vi "Registry - unregister silences appender.vi"(8 "error in (no error)":errorcluster) -> (0 "error out":errorcluster)   [LabVIEW 2026, in "Tests.lvlib"]
doc: "Verifies that unregistering one appender stops its delivery while the others keep receiving. Registers three queue-mode relay appenders, logs once (all three receive), unregisters relayB, logs again, and asserts the two survivors receive the second message and relayB receives nothing. Exercises the IDAbsent barrier in UnregisterAppender."
uses:
  Tests.lvlib
  src/TypeDefs/Severity.ctl
  <vilib>/addons/_JKI Toolkits/Caraya/classes/Assert/Assert False.vi
  <vilib>/addons/_JKI Toolkits/Caraya/classes/Assert/Assert Equal Value_Variant.vi
  <vilib>/addons/_JKI Toolkits/Caraya/classes/Assert/Assert True.vi
  <vilib>/addons/_JKI Toolkits/Caraya/classes/Assert/Assert Not Error.vi
  <vilib>/addons/_JKI Toolkits/Caraya/classes/Test/Test.lvclass
  src/Lumberjack.lvlib
  src/Public/Logger.lvclass/Logger.lvclass
  <vilib>/addons/_JKI Toolkits/Caraya/classes/Assert/Assert.lvclass
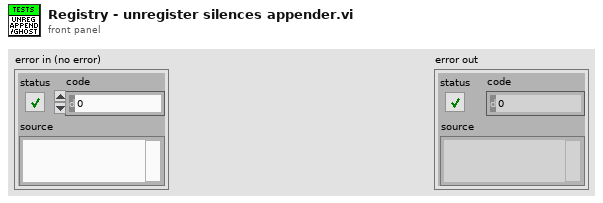
[diagram p1: front panel]
types:
  T1 = typedef "Lumberjack.lvlib/Severity.ctl" = enum16{"OFF", "FATAL", "ERROR", "WARN", "INFO", "DEBUG", "TRACE", "ALL"}
  T2 = typedef "Lumberjack.lvlib/Statement.ctl" = cluster{"timestamp":timestamp, "level":T1, "sourceTag":string, "originVI":string, "message":string}
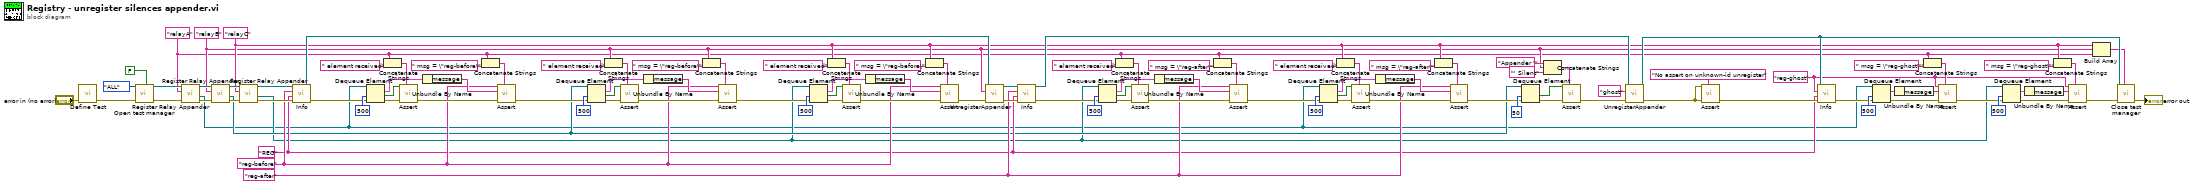
[diagram p0: block diagram]
diagram:
  w11 = "reg-ghost" ("message")
  w41 = "reg-after" ("message")
  w7 = "relayC"
  w6 = "relayB"
  w5 = "relayA"
  w27 = "REG" ("sourceTag")
  w68 = "reg-before" ("message")
  n1 = call <vilib>:"Define Test.vi"("error in (no error)"="error in (no error)") -> ("error out"=w111:errorcluster)  [unwired: 9 in, 1 out]
  n2 = call "Open test manager.vi"("enableDefaultFile"=FALSE, "error in (no error)"=w111, "globalThreshold"=Severity."ALL") -> ("error out"=w108:errorcluster, "Logger out"=w109:refnum<class "Logger.lvclass">)  [unwired: 7 in]
  n3 = call "Register Relay Appender.vi"("error in (no error)"=w108, "id in"=w5, "Logger in"=w109) -> ("error out"=w107:errorcluster, "relayQueue"=w3:refnum<queue>, "Logger out"=w106:refnum<class "Logger.lvclass">)  [unwired: 5 in, 1 out]
  n4 = call "Register Relay Appender.vi"("error in (no error)"=w107, "id in"=w6, "Logger in"=w106) -> ("error out"=w105:errorcluster, "relayQueue"=w8:refnum<queue>, "Logger out"=w104:refnum<class "Logger.lvclass">)  [unwired: 5 in, 1 out]
  n5 = call "Register Relay Appender.vi"("error in (no error)"=w105, "id in"=w7, "Logger in"=w104) -> ("error out"=w103:errorcluster, "relayQueue"=w4:refnum<queue>, "Logger out"=w102:refnum<class "Logger.lvclass">)  [unwired: 5 in, 1 out]
  n6 = call "Info.vi"("error in (no error)"=w103, "sourceTag"=w27, "message"=w68, "Logger in"=w102) -> ("error out"=w100:errorcluster, "Logger out"=w64:refnum<class "Logger.lvclass">)  [unwired: 6 in]
  n7 = Dequeue Element(queue=w3, timeout in ms (-1)=500, error in (no error)=w100) -> (element=w94:T2, timed out?=w93:bool, error out=w95:errorcluster)  [unwired: 1 out]
  n8 = Concatenate Strings(w5, " element received" ("Label")) -> (w98:string)
  n9 = call-poly <vilib>:"Assert.vi"("Label"=w98, "error in (no error)"=w95, "False?"=w93) -> ("error out"=w99:errorcluster)  [unwired: 7 in, 1 out]
  n10 = Unbundle By Name(w94) -> ("message"=w97:string)
  n11 = Concatenate Strings(w5, " msg = \"reg-before\"" ("Label")) -> (w96:string)
  n12 = call-poly <vilib>:"Assert.vi"("Label"=w96, "error in (no error)"=w99, "Actual"=w97, "Expected"=w68) -> ("error out"=w80:errorcluster)  [unwired: 6 in, 1 out]
  n13 = Dequeue Element(queue=w8, timeout in ms (-1)=500, error in (no error)=w80) -> (element=w84:T2, timed out?=w83:bool, error out=w85:errorcluster)  [unwired: 1 out]
  n14 = Concatenate Strings(w6, " element received" ("Label")) -> (w88:string)
  n15 = call-poly <vilib>:"Assert.vi"("Label"=w88, "error in (no error)"=w85, "False?"=w83) -> ("error out"=w89:errorcluster)  [unwired: 7 in, 1 out]
  n16 = Unbundle By Name(w84) -> ("message"=w87:string)
  n17 = Concatenate Strings(w6, " msg = \"reg-before\"" ("Label")) -> (w86:string)
  n18 = call-poly <vilib>:"Assert.vi"("Label"=w86, "error in (no error)"=w89, "Actual"=w87, "Expected"=w68) -> ("error out"=w69:errorcluster)  [unwired: 6 in, 1 out]
  n19 = Dequeue Element(queue=w4, timeout in ms (-1)=500, error in (no error)=w69) -> (element=w73:T2, timed out?=w72:bool, error out=w74:errorcluster)  [unwired: 1 out]
  n20 = Concatenate Strings(w7, " element received" ("Label")) -> (w77:string)
  n21 = call-poly <vilib>:"Assert.vi"("Label"=w77, "error in (no error)"=w74, "False?"=w72) -> ("error out"=w78:errorcluster)  [unwired: 7 in, 1 out]
  n22 = Unbundle By Name(w73) -> ("message"=w76:string)
  n23 = Concatenate Strings(w7, " msg = \"reg-before\"" ("Label")) -> (w75:string)
  n24 = call-poly <vilib>:"Assert.vi"("Label"=w75, "error in (no error)"=w78, "Actual"=w76, "Expected"=w68) -> ("error out"=w67:errorcluster)  [unwired: 6 in, 1 out]
  n25 = call "UnregisterAppender.vi"("error in (no error)"=w67, "id"=w6, "Logger in"=w64) -> ("error out"=w66:errorcluster, "Logger out"=w65:refnum<class "Logger.lvclass">)  [unwired: 7 in]
  n26 = call "Info.vi"("error in (no error)"=w66, "sourceTag"=w27, "message"=w41, "Logger in"=w65) -> ("error out"=w42:errorcluster, "Logger out"=w29:refnum<class "Logger.lvclass">)  [unwired: 6 in]
  n27 = Dequeue Element(queue=w4, timeout in ms (-1)=500, error in (no error)=w42) -> (element=w57:T2, timed out?=w56:bool, error out=w58:errorcluster)  [unwired: 1 out]
  n28 = Concatenate Strings(w5, " element received" ("Label")) -> (w61:string)
  n29 = call-poly <vilib>:"Assert.vi"("Label"=w61, "error in (no error)"=w58, "False?"=w56) -> ("error out"=w62:errorcluster)  [unwired: 7 in, 1 out]
  n30 = Unbundle By Name(w57) -> ("message"=w60:string)
  n31 = Concatenate Strings(w5, " msg = \"reg-after\"" ("Label")) -> (w59:string)
  n32 = call-poly <vilib>:"Assert.vi"("Label"=w59, "error in (no error)"=w62, "Actual"=w60, "Expected"=w41) -> ("error out"=w43:errorcluster)  [unwired: 6 in, 1 out]
  n33 = Dequeue Element(queue=w3, timeout in ms (-1)=500, error in (no error)=w43) -> (element=w47:T2, timed out?=w46:bool, error out=w48:errorcluster)  [unwired: 1 out]
  n34 = Concatenate Strings(w7, " element received" ("Label")) -> (w51:string)
  n35 = call-poly <vilib>:"Assert.vi"("Label"=w51, "error in (no error)"=w48, "False?"=w46) -> ("error out"=w52:errorcluster)  [unwired: 7 in, 1 out]
  n36 = Unbundle By Name(w47) -> ("message"=w50:string)
  n37 = Concatenate Strings(w7, " msg = \"reg-after\"" ("Label")) -> (w49:string)
  n38 = call-poly <vilib>:"Assert.vi"("Label"=w49, "error in (no error)"=w52, "Actual"=w50, "Expected"=w41) -> ("error out"=w34:errorcluster)  [unwired: 6 in, 1 out]
  n39 = Dequeue Element(queue=w8, timeout in ms (-1)=50, error in (no error)=w34) -> (timed out?=w38:bool, error out=w39:errorcluster)  [unwired: 2 out]
  n40 = Concatenate Strings("Appender '" ("string"), w6, "' Silent" ("Label")) -> (w35:string)
  n41 = call-poly <vilib>:"Assert.vi"("Label"=w35, "error in (no error)"=w39, "True?"=w38) -> ("error out"=w32:errorcluster)  [unwired: 7 in, 1 out]
  n42 = call "UnregisterAppender.vi"("error in (no error)"=w32, "id"="ghost", "Logger in"=w29) -> ("error out"=w26:errorcluster, "Logger out"=w28:refnum<class "Logger.lvclass">)  [unwired: 7 in]
  n43 = call-poly <vilib>:"Assert.vi"("Label"="No assert on unknown-id unregister", "error in (no error)"=w26, "Not Error?"=w26) -> ("error out"=w30:errorcluster)  [unwired: 7 in, 1 out]
  n44 = call "Info.vi"("error in (no error)"=w30, "sourceTag"=w27, "message"=w11, "Logger in"=w28) -> ("error out"=w21:errorcluster)  [unwired: 6 in, 1 out]
  n45 = Dequeue Element(queue=w3, timeout in ms (-1)=500, error in (no error)=w21) -> (element=w19:T2, error out=w20:errorcluster)  [unwired: 2 out]
  n46 = Unbundle By Name(w19) -> ("message"=w25:string)
  n47 = Concatenate Strings(w5, " msg = \"reg-ghost\"" ("Label")) -> (w24:string)
  n48 = call-poly <vilib>:"Assert.vi"("Label"=w24, "error in (no error)"=w20, "Actual"=w25, "Expected"=w11) -> ("error out"=w12:errorcluster)  [unwired: 6 in, 1 out]
  n49 = Dequeue Element(queue=w4, timeout in ms (-1)=500, error in (no error)=w12) -> (element=w13:T2, error out=w14:errorcluster)  [unwired: 2 out]
  n50 = Unbundle By Name(w13) -> ("message"=w18:string)
  n51 = Concatenate Strings(w7, " msg = \"reg-ghost\"" ("Label")) -> (w17:string)
  n52 = call-poly <vilib>:"Assert.vi"("Label"=w17, "error in (no error)"=w14, "Actual"=w18, "Expected"=w11) -> ("error out"=w10:errorcluster)  [unwired: 6 in, 1 out]
  n53 = Build Array(w7, w6, w5) -> (w2:string[])
  n54 = call "Close test manager.vi"("queueIDList"=w2, "error in (no error)"=w10, "Logger in"=w28) -> ("error out"=→"error out":errorcluster)  [unwired: 6 in]
